vi "labview proje ödevi1.vi"() -> ()   [LabVIEW 2017]
doc: "http://decibel.ni.com/content/docs/DOC-14442"
uses:
  <vilib>/Platform/browser.llb/Open URL in Default Browser (string).vi
panel:
  in  "Size":enum16{"Small", "Large", "Custom"}(ring)
  out "QR URL":string="http://chart.apis.google.com/chart?chs=500x500&cht=qr&chl=https://decibel.ni.com/content/docs/DOC-14442&choe=UTF-8&chld=L"
  in  "Error Correction Level":T1(ring)
  in  "Format Type":enum16{"UTF-8", "Shift_JIS", "ISO-8859-1"}(ring)
  in  "Data To Encode":string="https://decibel.ni.com/content/docs/DOC-14442"
  in  "CustomHeight":u16=500
  in  "Custom Width":u16=500
  # "QR Code Generator"
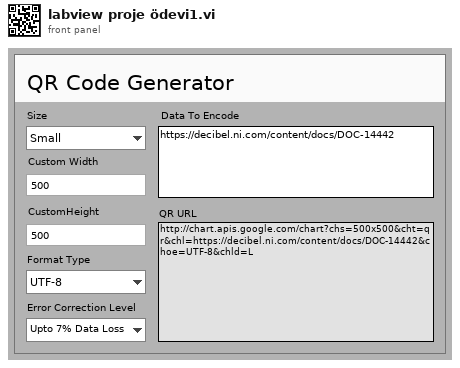
[diagram p1: front panel]
types:
  T1 = enum16{"Upto 7% Data Loss", "Upto 15% Data Loss", "Upto 25% Data Loss", "Upto 30% Data Loss"}
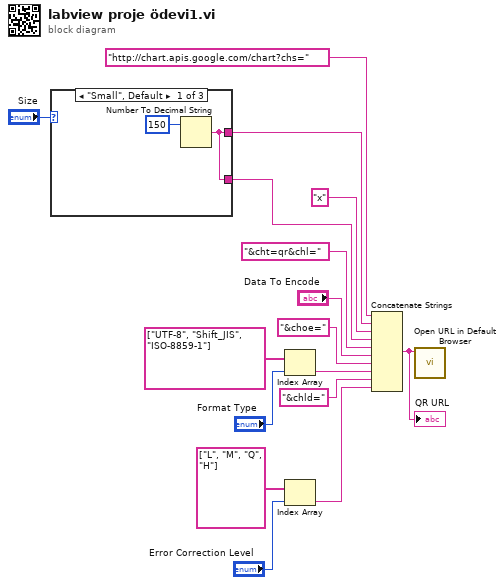
[diagram p0: block diagram]
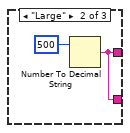
[diagram p2: hidden frame]
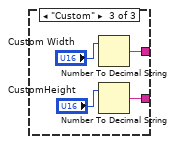
[diagram p3: hidden frame]
diagram:
  n1 = case shown="\"Small\", Default" "Size" {
    tunnel: [w17 w20 w22] -> w3
    tunnel: [w17 w20 w21] -> w2
    frame "Small", Default {
      n2 = Number To Decimal String(number=150) -> (decimal integer string=w17:string)  [unwired: 1 in]
    }
    frame "Large" {
      n3 = Number To Decimal String(number=500) -> (decimal integer string=w20:string)  [unwired: 1 in]
    }
    frame "Custom" {
      n4 = Number To Decimal String(number="Custom Width") -> (decimal integer string=w22:string)  [unwired: 1 in]
      n5 = Number To Decimal String(number="CustomHeight") -> (decimal integer string=w21:string)  [unwired: 1 in]
    }
  }
  n6 = Index Array(array=string[] ["UTF-8", "Shift_JIS", "ISO-8859-1"], index="Format Type") -> (element=w5:string)
  n7 = Index Array(array=string[] ["L", "M", "Q", "H"], index="Error Correction Level") -> (element=w8:string)
  n8 = Concatenate Strings("http://chart.apis.google.com/chart?chs=", w3, "x" ("string"), w2, "&cht=qr&chl=" ("string"), "Data To Encode", "&choe=" ("string"), w5, "&chld=" ("string"), w8) -> (w1:string)
  "QR URL" <- w1
  n9 = call-poly <vilib>:"Open URL in Default Browser.vi"("URL"=w1) -> ()  [unwired: 5 in, 2 out]
